vi "Drive Global Data.vi"() -> ()   [LabVIEW 2013]
panel:
  in  "Drive Global Data":T1
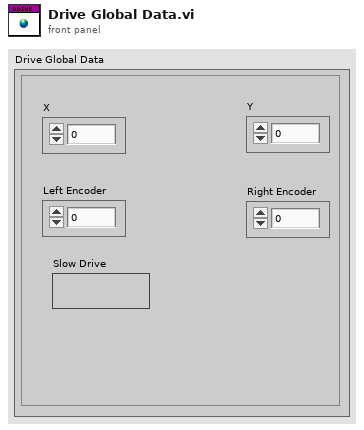
[diagram p1: front panel]
types:
  T1 = cluster{"Y":dbl, "X":dbl, "Left Encoder":dbl, "Right Encoder":dbl, "Slow Drive":bool}
diagram:
